vi "Read Data.vi"(7 "Instruction":T1=enum."Read Result", 8 "error in (no error)":errorcluster, 11 "connection ID":refnum<k5>) -> (0 "error out":errorcluster, 3 "connection ID out":refnum<k5>, 5 "Data":string)   [LabVIEW 2019, in "ACSVcontrol-driver.lvlib"]
doc: "Read data from TCP."
uses:
  ACSVcontrol-driver.lvlib
  Type definitions/Instruction.ctl
  Type definitions/Debug data.ctl
  Globals.vi
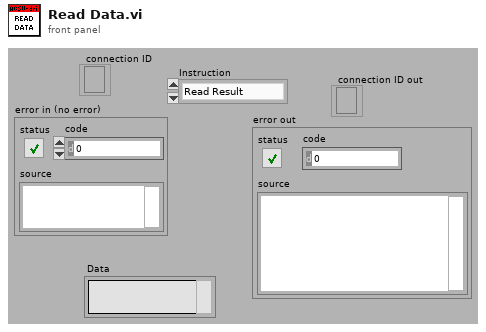
[diagram p1: front panel]
types:
  T1 = typedef "ACSVcontrol-driver.lvlib/Instruction.ctl" = enum16{"dummy - do not use", "Send Command", "Read Result", "Ask Status"}
  T2 = typedef "ACSVcontrol-driver.lvlib/Timeouts.ctl" = cluster{"TCP Read & Write (ms)":i32, "Sensors readout":i32, "PJVS setup":i32, "Nullmeter readout":i32, "Multiplexer setup":i32, "57XX setup":i32, "Generator setup":i32, "Synthesizer setup":i32, "Sampler readout":i32}
  T3 = typedef "ACSVcontrol-driver.lvlib/Debug data.ctl" = cluster{"Time Stamp":timestamp, "Data":string, "Write":bool, "Call chain":string[], "Error after":errorcluster}
  T4 = typedef "ACSVcontrol-driver.lvlib/Debug status.ctl" = enum16{"No change", "Off", "On"}
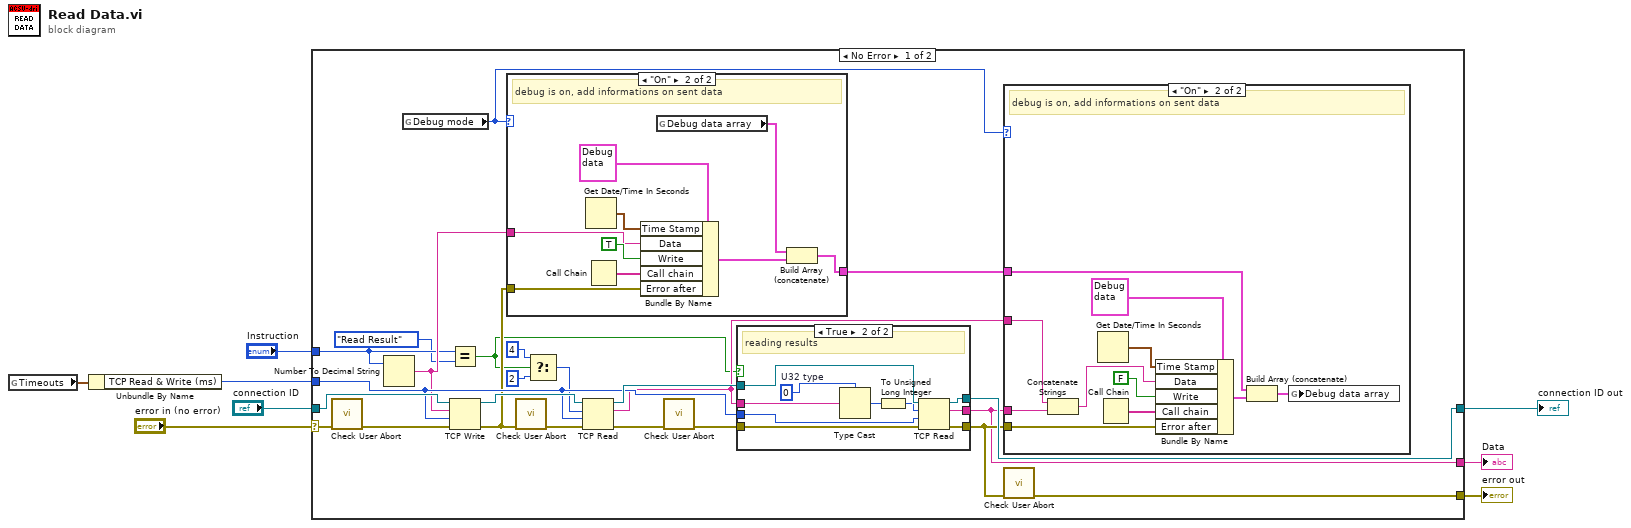
[diagram p0: block diagram]
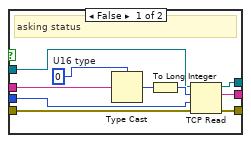
[diagram p2: hidden frame]
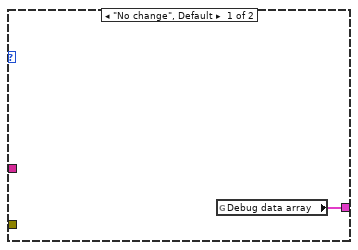
[diagram p4: hidden frame]
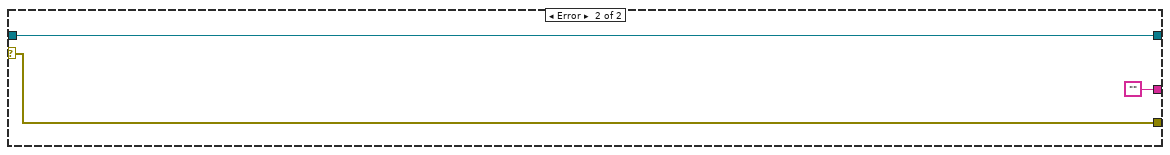
[diagram p5: hidden frame]
diagram:
  n1 = global read "Globals.vi" "Timeouts"() -> (w1:T2)
  n2 = Unbundle By Name(w1) -> ("TCP Read & Write (ms)"=w2:i32)
  n3 = case shown="No Error" "error in (no error)" {
    selector: "error in (no error)" -> [w23 w76]
    tunnel: [w29 w74] -> w6
    tunnel: [w24 w76] -> w7
    tunnel: "connection ID" -> [w30 w74]
    tunnel: w2 -> [w28 _]
    tunnel: [w15 ""] -> w4
    tunnel: "Instruction" -> [w14 _]
    frame No Error {
      n4 = call "Check User Abort.vi"("error in (no error)"=w23) -> ("error out"=w22:errorcluster)  [unwired: 10 in]
      n5 = Number To Decimal String(number=w14) -> (decimal integer string=w19:string)  [unwired: 1 in]
      n6 = global read "Globals.vi" "Debug mode"() -> (w21:T4)
      n7 = Equal?(x=w14, y=Instruction."Read Result") -> (x = y?=w9:bool)
      n8 = TCP Write(connection ID=w30, data in=w19, error in (no error)=w22, 9:w28) -> (connection ID out=w32:refnum<k5>, error out=w18:errorcluster)  [unwired: 1 out]
      n9 = case shown="\"On\"" w21 {
        tunnel: w18 -> [_ w67]
        tunnel: [w64 w66] -> w20
        tunnel: w19 -> [_ w65]
        frame "No change", Default {
          n10 = global read "Globals.vi" "Debug data array"() -> (w64:T3[])
        }
        frame "On" {
          # "debug is on, add informations on sent data"
          n11 = Get Date/Time In Seconds() -> (seconds since 1Jan1904=w72:timestamp)
          n12 = Call Chain() -> (call chain=w71:string[])
          n13 = Bundle By Name(cluster=T3 {"Time Stamp"=timestamp(0 s since 1904-01-01), "Data"="", "Write"=FALSE, "Call chain"=[], "Error after"={"status"=FALSE, "code"=0, "source"=""}} ("Debug data"), "Time Stamp"=w72, "Data"=w65, "Write"=TRUE ("Sent"), "Call chain"=w71, "Error after"=w67) -> (w68:T3)
          n14 = global read "Globals.vi" "Debug data array"() -> (w69:T3[])
          n15 = Build Array (concatenate)(w69, w68) -> (w66:T3[])
        }
      }
      n16 = call "Check User Abort.vi"("error in (no error)"=w18) -> ("error out"=w27:errorcluster)  [unwired: 10 in]
      n17 = Select(t=4 ("bytes to read"), s=w9, f=2 ("bytes to read")) -> (s? t:f=w11:i32)
      n18 = TCP Read(connection ID=w32, bytes to read=w11, error in (no error)=w27, 9:w28) -> (connection ID out=w31:refnum<k5>, data out=w16:string, error out=w26:errorcluster)  [unwired: 1 in]
      n19 = call "Check User Abort.vi"("error in (no error)"=w26) -> ("error out"=w25:errorcluster)  [unwired: 10 in]
      n20 = case shown="True" w9 {
        tunnel: w31 -> [w39 w52]
        tunnel: [w33 w48] -> w29
        tunnel: w28 -> [w38 w47]
        tunnel: w25 -> [w36 w46]
        tunnel: [w35 w45] -> w17
        tunnel: w16 -> [w37 w44]
        tunnel: [w34 w43] -> w15
        frame False {
          w40 = u16 0  # U16 type
          # "asking status"
          n21 = Type Cast(type=w40, x=w37) -> (*(type *) &x=w42:u16)
          n22 = To Long Integer(number=w42) -> (32bit integer=w41:i32)
          n23 = TCP Read(connection ID=w39, bytes to read=w41, error in (no error)=w36, 9:w38) -> (connection ID out=w33:refnum<k5>, data out=w34:string, error out=w35:errorcluster)  [unwired: 1 in]
        }
        frame True {
          w51 = u32 0  # U32 type
          # "reading results"
          n24 = Type Cast(type=w51, x=w44) -> (*(type *) &x=w50:u32)
          n25 = To Unsigned Long Integer(number=w50) -> (unsigned 32bit integer=w49:u32)
          n26 = TCP Read(connection ID=w52, bytes to read=w49, error in (no error)=w46, 9:w47) -> (connection ID out=w48:refnum<k5>, data out=w43:string, error out=w45:errorcluster)  [unwired: 1 in]
        }
      }
      n27 = case shown="\"On\"" w21 {
        tunnel: w17 -> [_ w57]
        tunnel: w20 -> [_ w56]
        tunnel: w16 -> [_ w54]
        tunnel: w15 -> [_ w53]
        frame "No change", Default {
        }
        frame "On" {
          # "debug is on, add informations on sent data"
          n28 = Concatenate Strings(w54, w53) -> (w55:string)
          n29 = Get Date/Time In Seconds() -> (seconds since 1Jan1904=w62:timestamp)
          n30 = Call Chain() -> (call chain=w61:string[])
          n31 = Bundle By Name(cluster=T3 {"Time Stamp"=timestamp(0 s since 1904-01-01), "Data"="", "Write"=FALSE, "Call chain"=[], "Error after"={"status"=FALSE, "code"=0, "source"=""}} ("Debug data"), "Time Stamp"=w62, "Data"=w55, "Write"=FALSE ("Sent"), "Call chain"=w61, "Error after"=w57) -> (w59:T3)
          n32 = Build Array (concatenate)(w56, w59) -> (w58:T3[])
          n33 = global write "Globals.vi" "Debug data array"(w58) -> ()
        }
      }
      n34 = call "Check User Abort.vi"("error in (no error)"=w17) -> ("error out"=w24:errorcluster)  [unwired: 10 in]
    }
    frame Error {
    }
  }
  "error out" <- w7
  "connection ID out" <- w6
  "Data" <- w4
